vi "AlignedArrayStack_subvi.vi"(8 "Window Length":i32, 9 "Peak Index":i32, 10 "Old Stack":dbl[][](array[numeric]), 11 "New Trace":dbl[](array[numeric])) -> (2 "New Stack":dbl[][](array[numeric]), 3 "Mini Window":dbl[](array[numeric]))   [LabVIEW 2019]
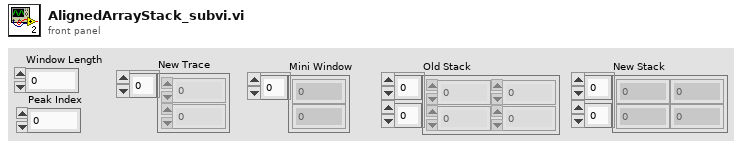
[diagram p1: front panel]
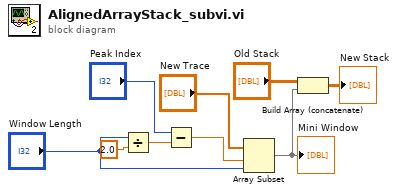
[diagram p0: block diagram]
diagram:
  n1 = Divide(x="Window Length", y=2.0) -> (x/y=w8:dbl)
  n2 = Subtract(x="Peak Index", y=w8) -> (x-y=w7:dbl)
  n3 = Array Subset(array="New Trace", index=w7, length="Window Length") -> (w3:dbl[])
  "Mini Window" <- w3
  n4 = Build Array (concatenate)("Old Stack", w3) -> (→"New Stack":dbl[][])
